vi "dscCounterDirectSet.vi"(6 "ctr_number":u8, 8 "error in":errorcluster, 9 "data":u32, 10 "code":u8, 11 "board":i16) -> (0 "error out":errorcluster, 3 "boardOut":i16)   [LabVIEW 2011, in "Diamond Universal Driver.lvlib"]
doc: "Sets the configuration for an individual counter on an 82C54 chip. Function provides direct access to the chip configuration register, enabling functionality other than simple rate generator. See data sheet for configuration data."
uses:
  Diamond Universal Driver.lvlib
  Controls/error codes.ctl
  Instruments/WL OPC/Support/dlls/dscud.dll
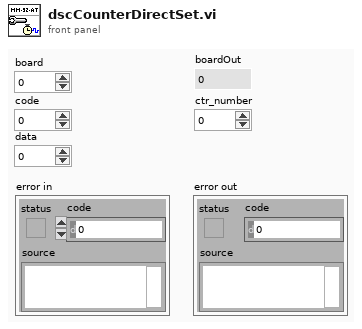
[diagram p1: front panel]
types:
  T1 = typedef "Diamond Universal Driver.lvlib/error codes.ctl" = enum8{"DE_NONE", "DE_HW_FAILURE", "DE_SW_FAILURE", "DE_HW_NOT_SUPPORTED", "DE_SW_NOT_SUPPORTED", "DE_INVALID_PARM", "DE_ALTERNATE_IN_PROGRESS", "DE_NONE_IN_PROGRESS", "DE_BUFFER_ROLLOVER", "DE_INVALID_ERROR_CODE", "DE_ALREADY_PAUSED", "DE_OVERFLOW", "DE_INVALID_FUNC", "DE_DSCUDH_INVALID", "DE_INVALID_BOARD", "DE_BOARD_LIMIT_REACHED", "DE_BOARD_BUSY", "DE_INVALID_WINDRVR_HANDLE", "DE_INVALID_WINDRVR_VERSION", "DE_BAD_WINDRVR_BOARD_INIT", "DE_OPERATION_TIMED_OUT", "DE_INVALID_WINDRVR_KP", "DE_THREAD_FAILURE"}
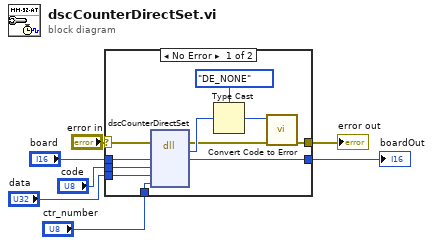
[diagram p0: block diagram]
diagram:
  n1 = case shown="No Error" "error in" {
    selector: "error in" -> [w18 w20]
    tunnel: [w14 w20] -> w6
    tunnel: [w12 w19] -> w5
    tunnel: "board" -> [w11 w19]
    tunnel: "code" -> [w10 _]
    tunnel: "data" -> [w9 _]
    tunnel: "ctr_number" -> [w8 _]
    frame No Error {
      n2 = dll-call lib="C:/Users/mrichardson/Documents/Web Based Version Control SW/Instruments/WL OPC/Support/dlls/dscud.dll" fn="dscCounterDirectSet"(error in=w18, "board"=w11, "code"=w10, "data"=w9, "ctr_number"=w8) -> (error out=w13:errorcluster, "error"=w17:u8, "board"=w12:i16)  [unwired: 5 in, 1 out]
      n3 = Type Cast(type=error_codes."DE_NONE" ("error codes"), x=w17) -> (*(type *) &x=w15:T1)
      n4 = call "Convert Code to Error.vi"("error in"=w13, "error codes"=w15) -> ("error out"=w14:errorcluster)  [unwired: 9 in]
    }
    frame Error {
    }
  }
  "error out" <- w6
  "boardOut" <- w5
